vi "Error Code to Error.vi"(11 "error code":i32) -> (0 "error":errorcluster)   [LabVIEW 2021]
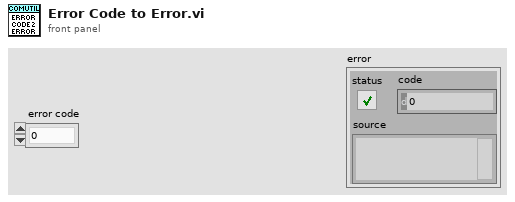
[diagram p1: front panel]
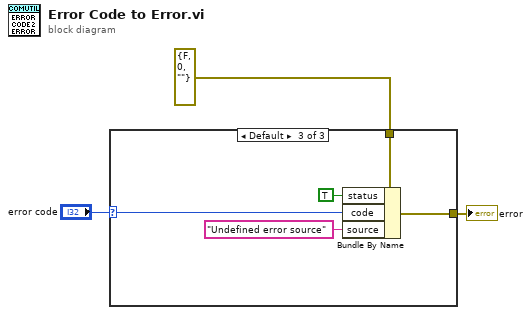
[diagram p0: block diagram]
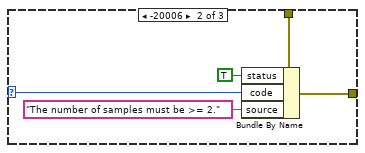
[diagram p3: hidden frame]
diagram:
  n1 = case shown="Default" "error code" {
    selector: "error code" -> [_ w8 w13]
    tunnel: errorcluster {"status"=FALSE, "code"=0, "source"=""} ("error constant") -> [w4 w9 w14]
    tunnel: [w4 w6 w11] -> w1
    frame 0.. {
    }
    frame -20006 {
      n2 = Bundle By Name(cluster=w9, "status"=TRUE, "code"=w8, "source"="The number of samples must be >= 2.") -> (w6:errorcluster)
    }
    frame Default {
      n3 = Bundle By Name(cluster=w14, "status"=TRUE, "code"=w13, "source"="Undefined error source") -> (w11:errorcluster)
    }
  }
  "error" <- w1
